vi "Execute.vi"(7 "Break at First Step? (F)":bool, 8 "error in (no error)":errorcluster, 11 "Execution in":refnum<class "Execution.lvclass">) -> (0 "error out":errorcluster, 3 "Execution out":refnum<class "Execution.lvclass">)   [LabVIEW 2020, in "TSnax.lvlib" / "Execution.lvclass"]
uses:
  Execution.lvclass
  Execution.lvclass/Execution.ctl
  PropertyObject/PropertyObject.lvclass/PropertyObject.ctl
  SequenceFile/SequenceFile.lvclass
  C:/dev/illuminated-g/tsnax/TSnax/PropertyObject/PropertyObject.lvclass
  PropertyObject/PropertyObject.lvclass
  Engine/Engine.lvclass
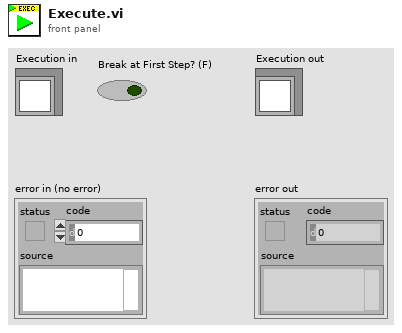
[diagram p1: front panel]
types:
  T1 = typedef "TSnax.lvlib/Execution.lvclass/Ref Data.ctl" = cluster{"Parameters":refnum<class "PropertyObject.lvclass">, "Client Sequence":refnum<class "SequenceFile.lvclass">, "Process Model":refnum<class "SequenceFile.lvclass">, "Entry Sequence":string, "Execution":refnum<k7>, "Report":refnum<class "Report.lvclass">, "Options":T2}
  T2 = typedef "TSnax.lvlib/Execution.lvclass/Execution Options.ctl" = cluster{"Use Default Model":bool, "Release Related References":bool}
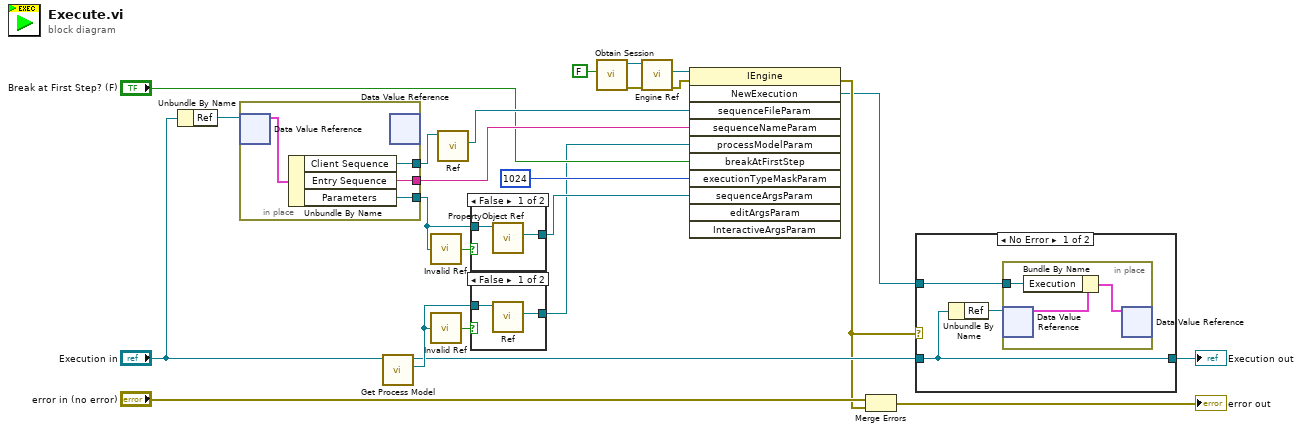
[diagram p0: block diagram]
diagram:
  n1 = Unbundle By Name("Execution in") -> ("Ref"=w23:refnum<data-value>)
  n2 = in-place {
    in-place-border: [w27] -> w15
    in-place-border: [w26] -> w13
    in-place-border: [w25] -> w21
    n3 = in-place-dvr #1(w23) -> (w28:T1)  [unwired: 1 out]
    n4 = Unbundle By Name(w28) -> ("Client Sequence"=w27:refnum<class "SequenceFile.lvclass">, "Entry Sequence"=w26:string, "Parameters"=w25:refnum<class "PropertyObject.lvclass">)
    n5 = in-place-dvr #1() -> ()  [unwired: 1 in, 2 out]
  }
  n6 = call "Get Process Model.vi"("Execution in"="Execution in") -> ("Process Model"=w7:refnum<class "SequenceFile.lvclass">, "Execution out"=w4:refnum<class "Execution.lvclass">)  [unwired: 8 in, 1 out]
  n7 = call "Invalid Ref.vi"("PropertyObject"=w21) -> ("Not a Valid Ref?"=w22:bool)
  n8 = call "Invalid Ref.vi"("PropertyObject"=w7) -> ("Not a Valid Ref?"=w8:bool)
  n9 = call "Ref.vi"("SequenceFile in"=w15) -> ("Ref"=w14:refnum<k7>)  [unwired: 8 in, 2 out]
  n10 = case shown="False" w22 {
    tunnel: w21 -> [w30 _]
    tunnel: [w29 _] -> w11
    frame False {
      n11 = call "PropertyObject Ref.vi"("PropertyObject in"=w30) -> ("PropertyObject"=w29:refnum<k7>)  [unwired: 8 in, 2 out]
    }
    frame True {
    }
  }
  n12 = case shown="False" w8 {
    tunnel: w7 -> [w32 _]
    tunnel: [w31 _] -> w6
    frame False {
      n13 = call "Ref.vi"("SequenceFile in"=w32) -> ("Ref"=w31:refnum<k7>)  [unwired: 8 in, 2 out]
    }
    frame True {
    }
  }
  n14 = call "Obtain Session.vi"("Create if needed? (T)"=FALSE) -> ("error out"=w18:errorcluster, "Engine out"=w20:refnum<class "Engine.lvclass">)  [unwired: 9 in]
  n15 = call "Engine Ref.vi"("error in (no error)"=w18, "Engine in"=w20) -> ("error out"=w17:errorcluster, "Engine"=w16:refnum<k7>)  [unwired: 7 in, 1 out]
  n16 = invoke class="IEngine" method="NewExecution"(reference=w16, error in=w17, "sequenceFileParam"=w14, "sequenceNameParam"=w13, "processModelParam"=w6, "breakAtFirstStep"="Break at First Step? (F)", "executionTypeMaskParam"=1024, "sequenceArgsParam"=w11) -> (error out=w3:errorcluster, "NewExecution"=w1:refnum<k7>)  [unwired: 3 in, 9 out]
  n17 = Merge Errors("error in (no error)", w3) -> (→"error out":errorcluster)
  n18 = case shown="No Error" w3 {
    tunnel: w4 -> [w34 w39]
    tunnel: [w34 w39] -> w2
    tunnel: w1 -> [w33 _]
    frame No Error {
      n19 = Unbundle By Name(w34) -> ("Ref"=w35:refnum<data-value>)
      n20 = in-place {
        in-place-border: w33 -> [w36]
        n21 = in-place-dvr #2(w35) -> (w38:T1)  [unwired: 1 out]
        n22 = Bundle By Name(cluster=w38, "Execution"=w36) -> (w37:T1)
        n23 = in-place-dvr #2(w37) -> ()  [unwired: 2 out]
      }
    }
    frame Error {
    }
  }
  "Execution out" <- w2
